vi "Configure Control Mode.vi"(8 "error in (no error)":errorcluster, 10 "control mode":u16(ring) items=["stop", "normal", "auto tuning", "learning", "external tune"], 11 "HECR in":refnum<class "PL SMC HECR.lvclass">) -> (0 "error out":errorcluster, 3 "HECR out":refnum<class "PL SMC HECR.lvclass">)   [LabVIEW 2015, in "PL SMC HECR.lvclass"]
doc: "Configures control mode."
uses:
  PL SMC HECR.lvclass
  <vilib>/plasmapper/PL Modbus Client/PL Modbus Client.lvclass
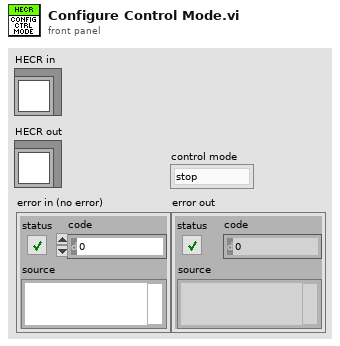
[diagram p1: front panel]
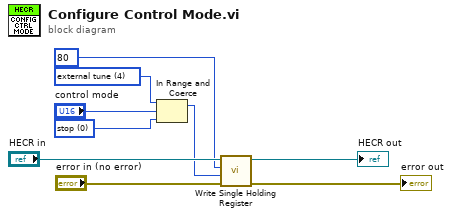
[diagram p0: block diagram]
diagram:
  w2 = u16 4 items=["stop", "normal", "auto tuning", "learning", "external tune"] ("mode")
  w1 = u16 0 items=["stop", "normal", "auto tuning", "learning", "external tune"] ("mode")
  n1 = In Range and Coerce(upper limit=w2, x="control mode", lower limit=w1) -> (coerced(x)=w4:u16)  [unwired: 1 out]
  n2 = call <vilib>:"Write Single Holding Register.vi"("error in (no error)"="error in (no error)", "value"=w4, "address"=u16 80, "MODBUS in"="HECR in") -> ("error out"=→"error out":errorcluster, "MODBUS out"=→"HECR out":refnum<class "PL SMC HECR.lvclass">)  [unwired: 6 in]
